vi "Do.vi"(8 "error in (no error)":errorcluster, 10 "Actor in":refnum<class "Actor.lvclass">, 11 "Update Fan Msg":refnum<class "Update Fan Msg.lvclass">) -> (0 "error out":errorcluster, 2 "Actor out":refnum<class "Actor.lvclass">)   [LabVIEW 2011, in "Cooler UI.lvlib" / "Update Fan Msg.lvclass"]
uses:
  Update Fan Msg.lvclass
  <vilib>/ActorFramework/Actor/Actor.lvclass
  Cooler UI with Events/Cooler UI with Events.lvclass
  Update Fan Msg.lvclass/Update Fan Msg.ctl
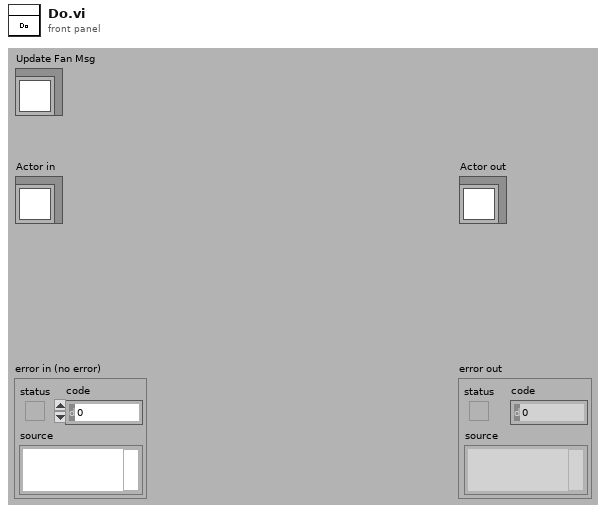
[diagram p1: front panel]
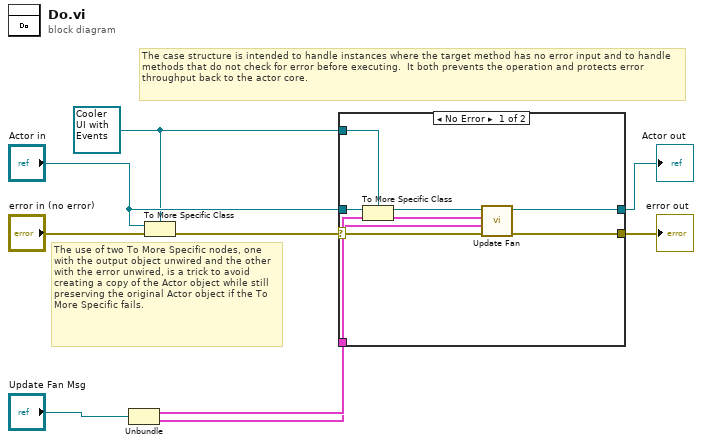
[diagram p0: block diagram]
diagram:
  w3 = refnum<class "Cooler UI with Events.lvclass"> refnum ("Actor in")
  # "The use of two To More Specific nodes, one with the output object unwired and the other with the error unwired, is a trick to avoid creating a copy of the Actor object while still preserving the original Actor object if the To More Specific fails."
  # "The case structure is intended to handle instances where the target method has no error input and to handle methods that do not check for error before executing.  It both prevents the operation and protects error throughput back to the actor core."
  n1 = Unbundle("Update Fan Msg") -> (w2:cluster{"State":bool, "Fault":bool}, w1:cluster{"State":bool, "Fault":bool})
  n2 = To More Specific Class(target class=w3, reference="Actor in", error in="error in (no error)") -> (error out=w7:errorcluster)  [unwired: 1 out]
  n3 = case shown="No Error" w7 {
    selector: w7 -> [w15 w19]
    tunnel: [w17 w19] -> w6
    tunnel: [w16 w18] -> w5
    tunnel: "Actor in" -> [w14 w18]
    tunnel: w3 -> [w13 _]
    tunnel: w2 -> [w11 _]
    tunnel: w1 -> [w10 _]
    frame No Error {
      n4 = To More Specific Class(target class=w13, reference=w14) -> (specific class reference=w12:refnum<class "Cooler UI with Events.lvclass">)  [unwired: 1 in, 1 out]
      n5 = call-dynamic "Update Fan.vi"("error in (no error)"=w15, "Fan B"=w10, "Fan A"=w11, "Cooler UI in"=w12) -> ("error out"=w17:errorcluster, "Cooler UI out"=w16:refnum<class "Cooler UI with Events.lvclass">)  [unwired: 6 in]
    }
    frame Error {
      # "If type check fails, pass the original object out again."
    }
  }
  "error out" <- w6
  "Actor out" <- w5
